vi "Example 32bit.vi"() -> ()   [LabVIEW 2019]
uses:
  Builds/32 bit/Menu Launcher Module.lvlibp
panel:
  in  "Position":T1(ring)
  out "Selected Options":string
  in  "Stop":bool
  in  "Menu":bool
  in  "Path":path
  # "1. Select Menu File in the menu file path\n2. Run the VI\n3. Select Menu Option to Launch SyncSols Menu\n4. Stop the VI using stop function"
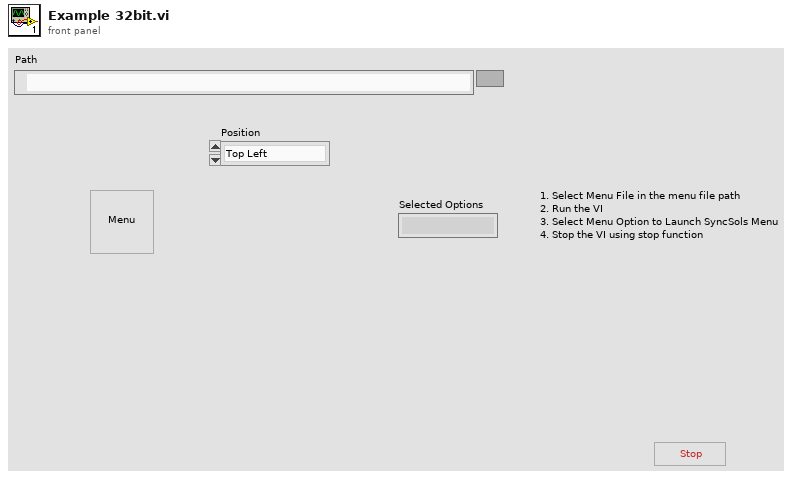
[diagram p1: front panel]
types:
  T1 = enum16{"Top Left", "Top Right", "Bottom Left", "Bottom Right", "Center"}
  T2 = typedef "Menu Launcher Module.lvlibp/Broadcast Events--cluster.ctl" = cluster{"Module Did Init":refnum<user-event>, "Status Updated":refnum<user-event>, "Error Reported":refnum<user-event>, "Module Did Stop":refnum<user-event>, "Update Module Execution Status":refnum<user-event>, "Get Selected Option":refnum<user-event>}
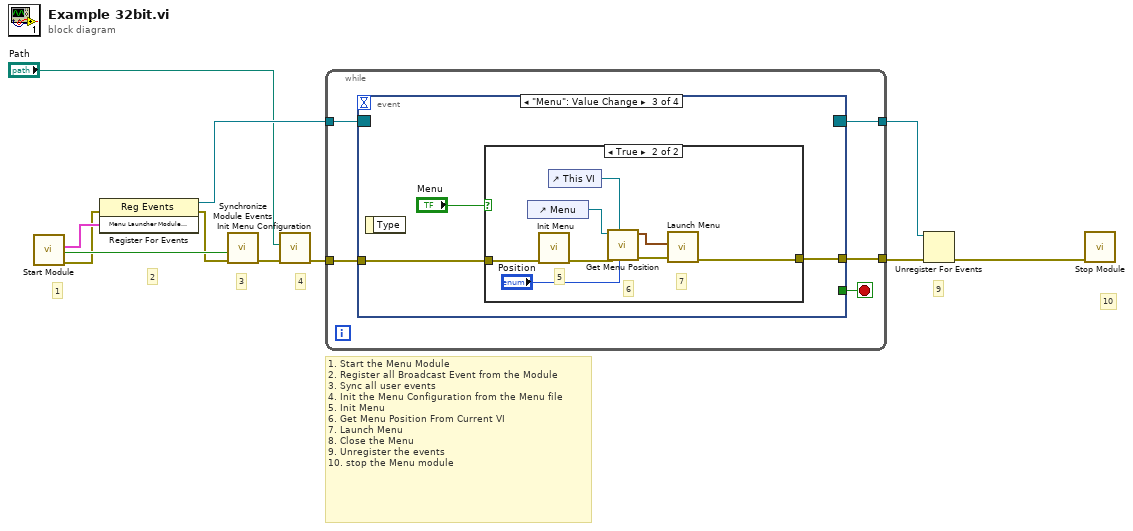
[diagram p0: block diagram]
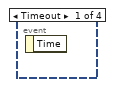
[diagram p2: hidden frame]
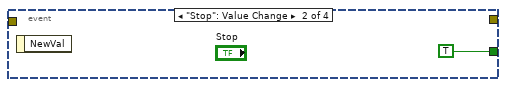
[diagram p3: hidden frame]
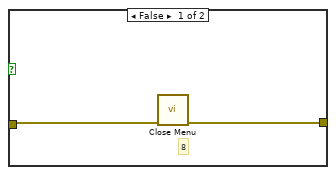
[diagram p4: hidden frame]
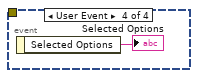
[diagram p5: hidden frame]
diagram:
  # "10"
  # "9"
  # "4"
  # "3"
  # "2"
  # "1"
  # "1. Start the Menu Module\n2. Register all Broadcast Event from the Module\n3. Sync all user events \n4. Init the Menu Configuration from the Menu file\n5. Init Menu\n6. Get Menu Position From Current VI\n7. Launch Menu\n8. Close the Menu\n9. Unregister the events\n10. stop the Menu module"
  n1 = call "Start Module.vi"() -> ("error out"=w8:errorcluster, "Wait for Event Sync?"=w10:bool, "Menu Launcher Module Broadcast Events"=w11:T2)  [unwired: 8 in, 1 out]
  n2 = register-events(error in=w8, w11) -> (reference out=w9:refnum<event-registration>, error out=w7:errorcluster)  [unwired: 1 in]
  n3 = call "Synchronize Module Events.vi"("error in (no error)"=w7, "Wait for Event Sync?"=w10) -> ("error out"=w5:errorcluster)  [unwired: 9 in]
  n4 = call "Init Menu Configuration.vi"("error in (no error)"=w5, "Menu File Path"="Path") -> ("error out"=w4:errorcluster)  [unwired: 9 in]
  n5 = while {
    tunnel: w4 -> [w15]
    tunnel: w9 -> [w16]
    tunnel: [w13] -> w3
    tunnel: [w12] -> w2
    stop <- w14 stop-if-true
    n6 = event shown="[2] \"Menu\": Value Change" {
      selector: w16 -> [_ _ _ _]
      dyn-events: [_ _ _ _] -> w12
      timeout: _ -> [_ _ _ _]
      tunnel: w15 -> [_ _ w19 _]
      tunnel: [_ TRUE _ _] -> w14
      tunnel: [_ _ w18 _] -> w13
      event Timeout {
        n7 = event-data() -> ()  [unwired: 1 in, 1 out]
      }
      event "Stop": Value Change {
        n8 = event-data() -> ()  [unwired: 1 in, 1 out]
      }
      event "Menu": Value Change {
        n9 = event-data() -> ()  [unwired: 1 in, 1 out]
        n10 = case shown="True" "Menu" {
          tunnel: w19 -> [w22 w25]
          tunnel: [w21 w24] -> w18
          frame False {
            # "8"
            n11 = call "Close Menu.vi"("error in (no error)"=w22) -> ("error out"=w21:errorcluster)  [unwired: 10 in]
          }
          frame True {
            # "7"
            # "6"
            # "5"
            n12 = control-ref of="Menu"() -> (w26:refnum<vi>)
            n13 = call "Init Menu.vi"("error in (no error)"=w25) -> ("error out"=w29:errorcluster)  [unwired: 10 in]
            n14 = control-ref of="This VI"() -> (w27:refnum<vi>)
            n15 = call "Get Menu Position.vi"("Position"="Position", "VI Refnum(Calling VI)"=w27, "error in (no error)"=w29, "Menu Refnum"=w26) -> ("error out"=w30:errorcluster, "Position"=w28:cluster{"Top":i16, "Left":i16})  [unwired: 6 in]
            n16 = call "Launch Menu.vi"("error in (no error)"=w30, "Position"=w28) -> ("error out"=w24:errorcluster)  [unwired: 9 in]
          }
        }
      }
      event User Event {
        n17 = event-data() -> ("Selected Options"=→"Selected Options":string)  [unwired: 1 in]
      }
    }
  }
  n18 = Unregister For Events(event registration refnum=w2, error in=w3) -> (error out=w1:errorcluster)
  n19 = call "Stop Module.vi"("error in (no error)"=w1) -> ()  [unwired: 10 in, 1 out]
